vi "Write VeriSTAND Channel Info.vi"(8 "error in (no error)":errorcluster, 9 "VeriSTAND Reference":T1=18446744073709551615 format="%.0x", 10 "Exist in VeriSTAND":bool, 11 "ChannelVS in":refnum<class "ChannelVS.lvclass">) -> (0 "error out":errorcluster, 3 "ChannelVS out":refnum<class "ChannelVS.lvclass">)   [LabVIEW 2017, in "Shared Variables CD 2.0 Configuration.lvlib" / "ChannelVS.lvclass"]
uses:
  ChannelVS.lvclass
  <vilib>/NI Veristand/Custom Device API/Custom Device Item Ref.ctl
  ChannelVS.lvclass/ChannelVS.ctl
  <vilib>/NI VeriStand/Custom Device API/Custom Device API.lvlib
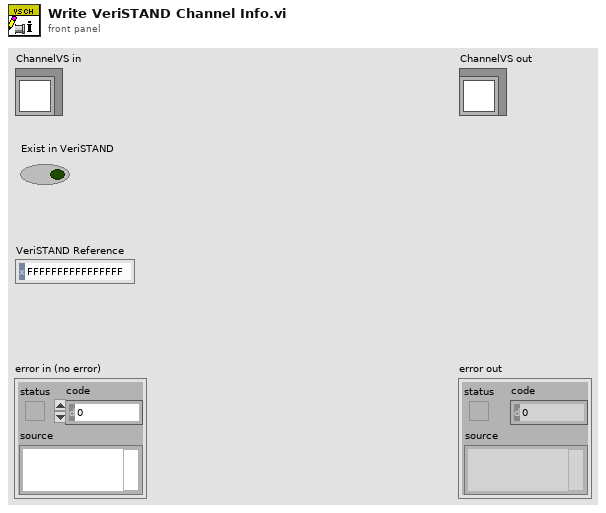
[diagram p1: front panel]
types:
  T1 = typedef "Custom Device API.lvlib/Custom Device Item Ref.ctl" = u64
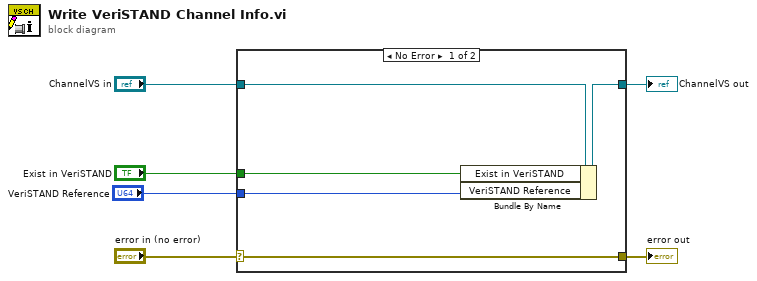
[diagram p0: block diagram]
diagram:
  n1 = case shown="No Error" "error in (no error)" {
    selector: "error in (no error)" -> [w11 w12]
    tunnel: [w11 w12] -> w5
    tunnel: [w9 w13] -> w3
    tunnel: "ChannelVS in" -> [w10 w13]
    tunnel: "Exist in VeriSTAND" -> [w8 _]
    tunnel: "VeriSTAND Reference" -> [w7 _]
    frame No Error {
      n2 = Bundle By Name(cluster=w10, "Exist in VeriSTAND"=w8, "VeriSTAND Reference"=w7) -> (w9:refnum<class "ChannelVS.lvclass">)
    }
    frame Error {
    }
  }
  "error out" <- w5
  "ChannelVS out" <- w3
